vi "TransducerFormulaCalc.vi"(1 "X":dbl, 2 "公式参数":dbl[](array[numeric])) -> (0 "Y":dbl)   [LabVIEW 2011]
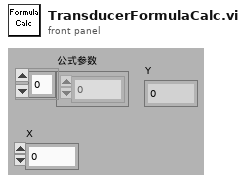
[diagram p1: front panel]
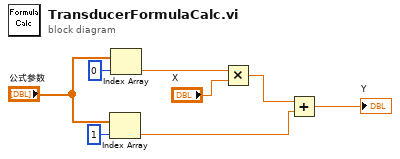
[diagram p0: block diagram]
diagram:
  n1 = Index Array(array="公式参数", index=1) -> (element=w1:dbl)
  n2 = Index Array(array="公式参数", index=0) -> (element=w2:dbl)
  n3 = Multiply(x=w2, y="X") -> (x*y=w7:dbl)
  n4 = Add(x=w7, y=w1) -> (x+y=→"Y":dbl)
